vi "Generate Sound.vi"() -> ()   [LabVIEW 2010]
doc: "This VI illustrates how to generate and play sine, square, sawtooth and triangle waveforms. You can change the frequency and type of the waveform generated as it plays continuously."
uses:
  <vilib>/sound2/lvsound2.llb/Sound Data Format.ctl
  <vilib>/sound2/lvsound2.llb/Sampling Mode.ctl
  <vilib>/sound2/lvsound2.llb/Sound Output Set Volume (Single).vi
  <vilib>/sound2/lvsound2.llb/Sound Output Write (DBL Single).vi
  <vilib>/measure/NI_MABase.lvlib
panel:
  out "millisecond timer value 2":u32
  out "Waveform Chart":sgl(graph)
  in  "Sound Format":T1={"sample rate (S/s)"=44100.0, "number of channels"=2, "bits per sample"=16}
  in  "Volume":dbl(slide)=70.40816326530613 scale=0.0..100.0
  out "Generated Sound":waveform(dbl)(graph)={"t0"=timestamp(1.2471655328798186 s since 1904-01-01), "dt"=2.2675736961451248e-05, "Y"=[]}
  in  "Waveform Type":enum16{"Sine", "Square", "Sawtooth", "Triangle"}(ring)
  in  "Frequency":dbl=500.0 format="%0.2p"
  in  "stop":bool
  in  "Number of Samples/ch":i32=5000
  in  "Device ID":u32
  # "This VI illustrates how to generate and play sine, square, sawtooth and triangle waveforms continuously. \n\nInstructions to execute the VI:\n1.  Specify Device ID, bits per sample, sample rate and number of samples (buffer size).\n2.  Select the waveform type to play and its initial frequency.\n3.  Run the VI. Waveforms are generated and sent to both the graph and your speakers.\n3.  Change the frequency to change the pitch of the sound.\n4.  Change the waveform type to start playing differently shaped waves.\n5.  Press the stop button when done."
  # "Configuration"
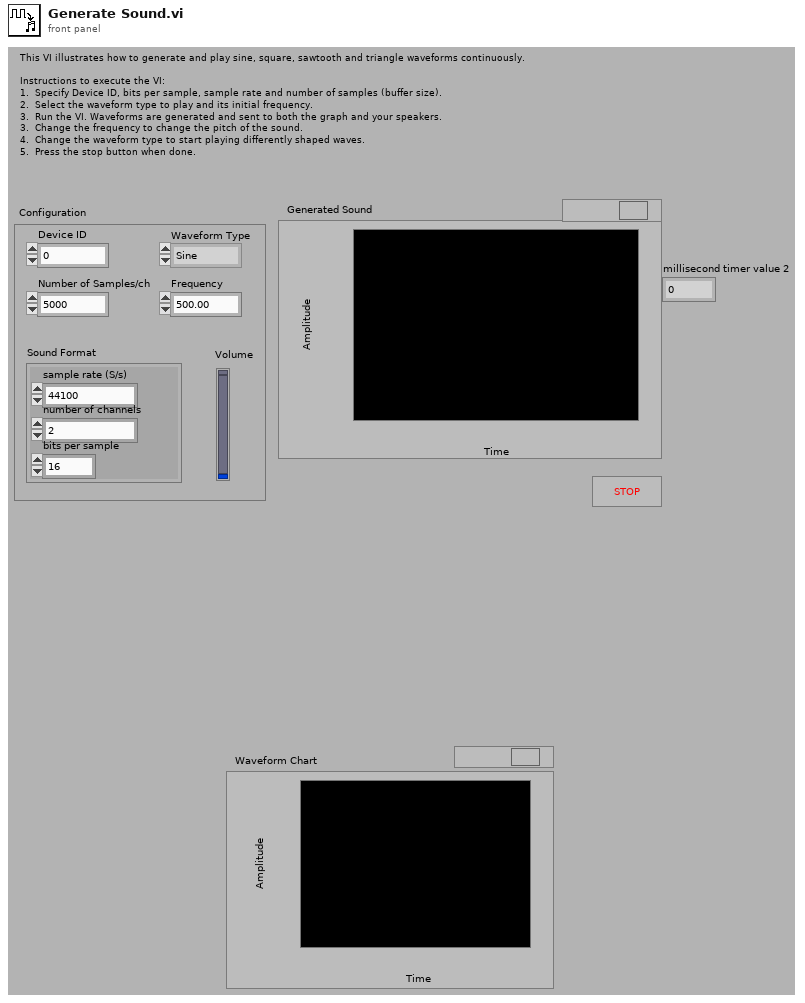
[diagram p1: front panel]
types:
  T1 = typedef "Sound Data Format.ctl" = cluster{"sample rate (S/s)":dbl, "number of channels":i32, "bits per sample":i32}
  T2 = typedef "Sampling Mode.ctl" = i32
  T3 = typedef "Sound Output Task ID.ctl" = u32
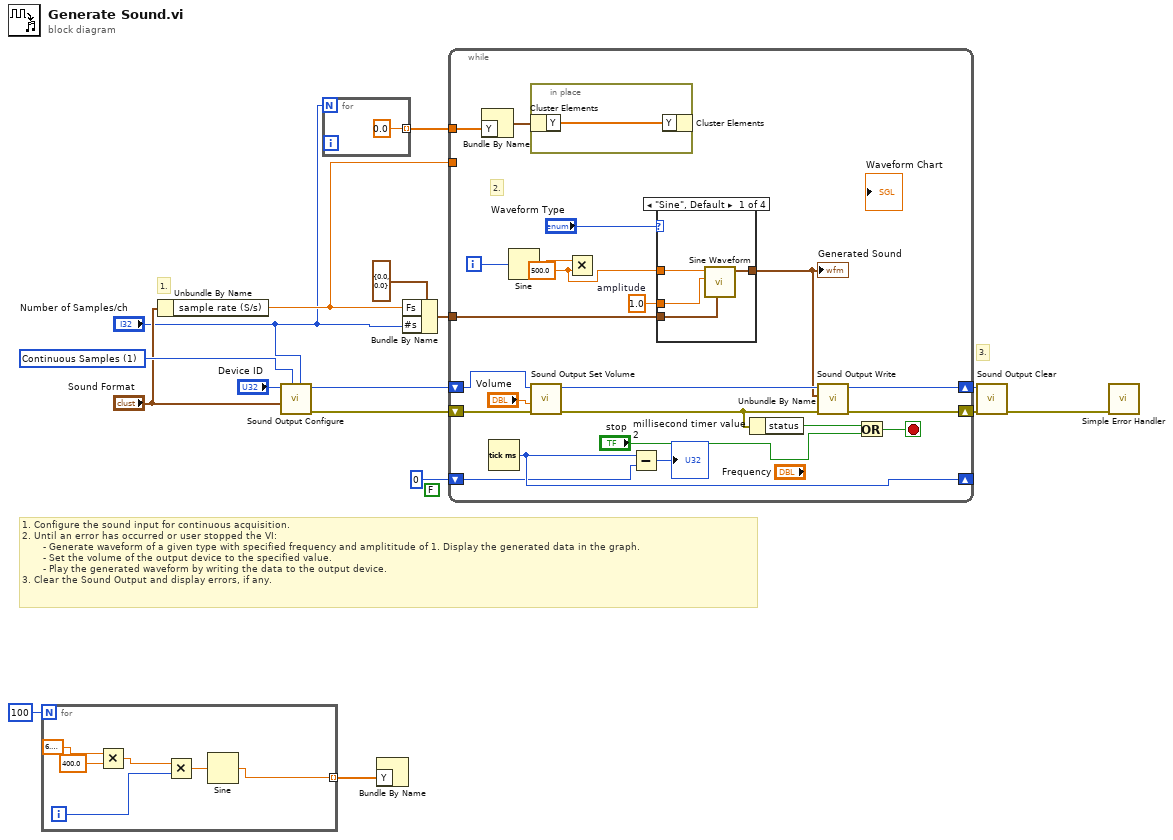
[diagram p0: block diagram]
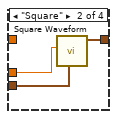
[diagram p2: hidden frame]
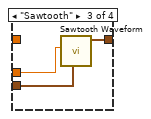
[diagram p3: hidden frame]
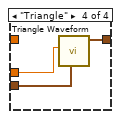
[diagram p4: hidden frame]
diagram:
  (unwired) FALSE
  w11 = T2 1 items=["Finite Samples", "Continuous Samples"] ("sample mode")
  # "3."
  # "1."
  # "1. Configure the sound input for continuous acquisition.\n2. Until an error has occurred or user stopped the VI: \n      \t- Generate waveform of a given type with specified frequency and amplititude of 1. Display the generated data in the graph. \n       - Set the volume of the output device to the specified value.\n      \t- Play the generated waveform by writing the data to the output device.\n3. Clear the Sound Output and display errors, if any."
  n1 = for {
    N: 100 -> [_]
    tunnel: [w19] -> w4 mode=indexing
    i -> [w17]
    n2 = Multiply(x=6.283185307179586, y=400.0) -> (x*y=w21:dbl)
    n3 = Multiply(x=w21, y=w17) -> (x*y=w20:dbl)
    n4 = Sine(x=w20) -> (sin(x)=w19:dbl)
  }
  n5 = Unbundle By Name("Sound Format") -> ("sample rate (S/s)"=w2:dbl)
  n6 = call <vilib>:"Sound Output Configure.vi"("number of samples/ch"="Number of Samples/ch", "sample mode"=w11, "sound format"="Sound Format", "device ID"="Device ID") -> ("error out"=w16:errorcluster, "task ID"=w15:T3)  [unwired: 6 in]
  n7 = for {
    N: "Number of Samples/ch" -> [_]
    tunnel: [0.0] -> w6 mode=indexing
  }
  n8 = Bundle By Name("Y"=w4) -> ()  [unwired: 1 in, 1 out]
  n9 = Bundle By Name(cluster=cluster{"Fs":dbl, "#s":dbl} {"Fs"=0.0, "#s"=0.0} ("sampling info"), "Fs"=w2, "#s"="Number of Samples/ch") -> (w9:cluster{"Fs":dbl, "#s":dbl})
  n10 = while {
    shift-right: [w44] -> w14
    shift-left: w16 -> [w39]
    shift-right: [w45] -> w13
    shift-left: w15 -> [w37]
    tunnel: w9 -> [w42]
    tunnel: w6 -> [w34]
    tunnel: w2 -> [_]
    shift-right: [w25] -> _
    shift-left: u32 0 ("millisecond timer value") -> [w24]
    i -> [w35]
    stop <- w27 stop-if-true
    w29 = 500.0 ("y")
    w41 = 1.0  # amplitude
    # "2."
    n11 = Bundle By Name("Y"=w34) -> (w33:waveform(dbl))  [unwired: 1 in]
    n12 = Tick Count (ms)() -> (millisecond timer value=w25:u32)
    n13 = Sine(x=w35) -> (sin(x)=w30:dbl)
    n14 = in-place {
      n15 = in-place-cluster #1(w33) -> ("Y"=w46:dbl[])
      n16 = in-place-cluster #1("Y"=w46) -> ()  [unwired: 1 out]
    }
    n17 = call-poly <vilib>:"Sound Output Set Volume.vi"("error in (no error)"=w39, "volume"="Volume", "task ID"=w37) -> ("error out"=w40:errorcluster, "task ID out"=w38:T3)  [unwired: 7 in]
    n18 = Multiply(x=w30, y=w29) -> ()  [unwired: 1 out]
    n19 = Subtract(x=w25, y=w24) -> (x-y=→"millisecond timer value 2":u32)
    n20 = case shown="\"Sine\", Default" "Waveform Type" {
      tunnel: [w50 w52 w55 w59] -> w32
      tunnel: w42 -> [w49 w53 w56 w58]
      tunnel: w41 -> [w48 w51 w54 w57]
      tunnel: w29 -> [w47 _ _ _]
      frame "Sine", Default {
        n21 = call <vilib>:"Sine Waveform.vi"("sampling info"=w49, "amplitude"=w48, "frequency"=w47) -> ("signal out"=w50:waveform(dbl))  [unwired: 7 in, 1 out]
      }
      frame "Square" {
        n22 = call <vilib>:"Square Waveform.vi"("sampling info"=w53, "amplitude"=w51) -> ("signal out"=w52:waveform(dbl))  [unwired: 8 in, 1 out]
      }
      frame "Sawtooth" {
        n23 = call <vilib>:"Sawtooth Waveform.vi"("sampling info"=w56, "amplitude"=w54) -> ("signal out"=w55:waveform(dbl))  [unwired: 8 in, 1 out]
      }
      frame "Triangle" {
        n24 = call <vilib>:"Triangle Waveform.vi"("sampling info"=w58, "amplitude"=w57) -> ("signal out"=w59:waveform(dbl))  [unwired: 8 in, 1 out]
      }
    }
    "Generated Sound" <- w32
    n25 = Unbundle By Name(w40) -> ("status"=w43:bool)
    n26 = call-poly <vilib>:"Sound Output Write.vi"("error in (no error)"=w40, "data"=w32, "task ID"=w38) -> ("error out"=w44:errorcluster, "task ID out"=w45:T3)  [unwired: 7 in]
    n27 = Or(x=w43, y="stop") -> (x .or. y?=w27:bool)
  }
  n28 = call <vilib>:"Sound Output Clear.vi"("error in (no error)"=w14, "task ID"=w13) -> ("error out"=w8:errorcluster)  [unwired: 9 in]
  n29 = call <vilib>:"Simple Error Handler.vi"("error in (no error)"=w8) -> ()  [unwired: 4 in, 5 out]
